vi "ejercicio 3.vi"() -> ()   [LabVIEW 2017]
panel:
  out "numero mayor en renglon":i64[](array[numeric])
  out "suma columnas":i64[](array[numeric])
  out "suma filas":i64[](array[numeric])
  out "renglon\nmax suma":i64
  out "columna\nmax suma":i64
  out "numero mayor\nrenglon 10":i64
  out "numero mayor\nrenglon 9":i64
  out "numero mayor\nrenglon 8":i64
  out "numero mayor\nrenglon 7":i64
  out "numero mayor\nrenglon 6":i64
  out "numero mayor\nrenglon 5":i64
  out "numero mayor\nrenglon 4":i64
  out "numero mayor\nrenglon 3":i64
  out "numero mayor\nrenglon 2":i64
  out "numero mayor\nrenglon 1":i64
  out "Max":i64
  out "Arreglo":i64[][](array[numeric])
  # "Ejercicio 3\nDiseñe un programa que llene una matriz de 10 x 10 y determine:\nEl numero mayor almacenado en la matriz\nEl numero mayor almacenado en cada renglon\nLa columna que tuvo la maxima suma\nEl renglon que tuvo la maxima suma"
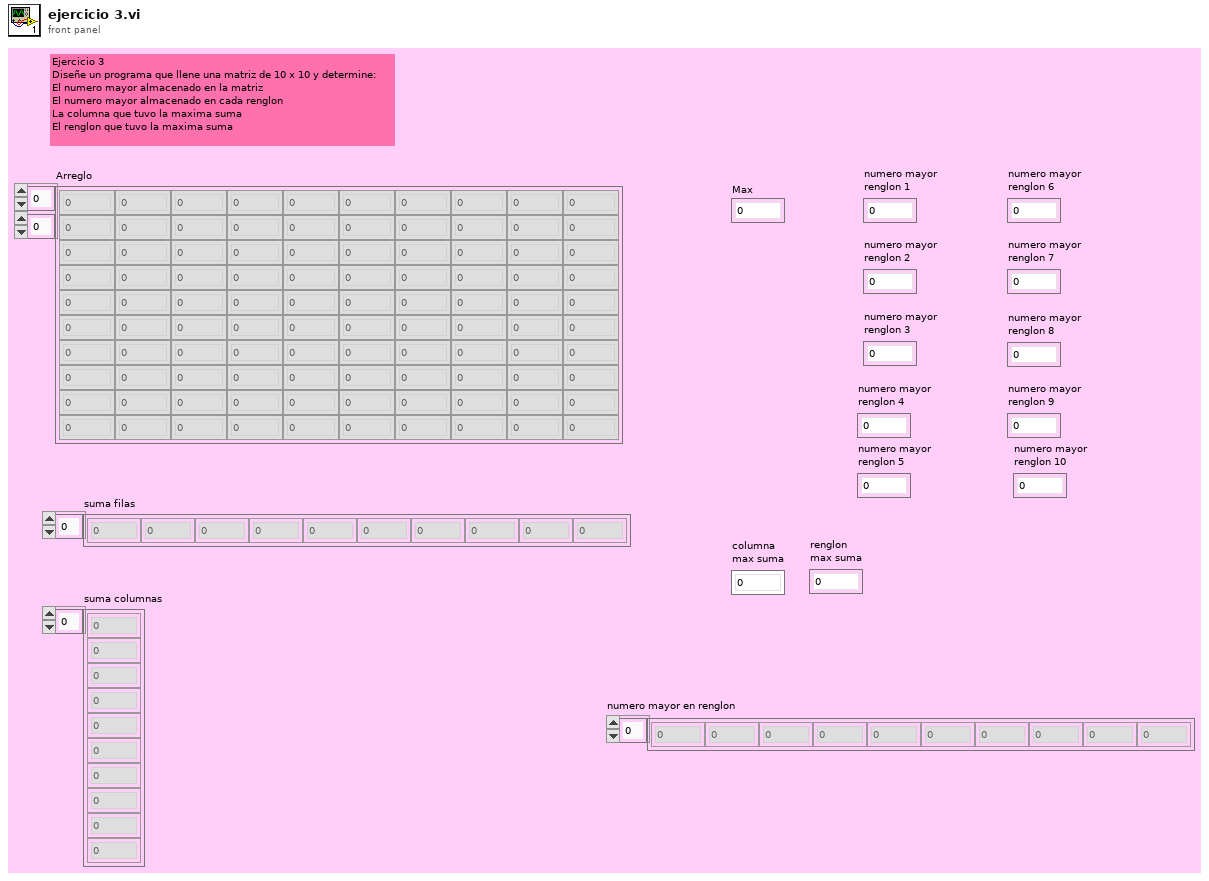
[diagram p1: front panel]
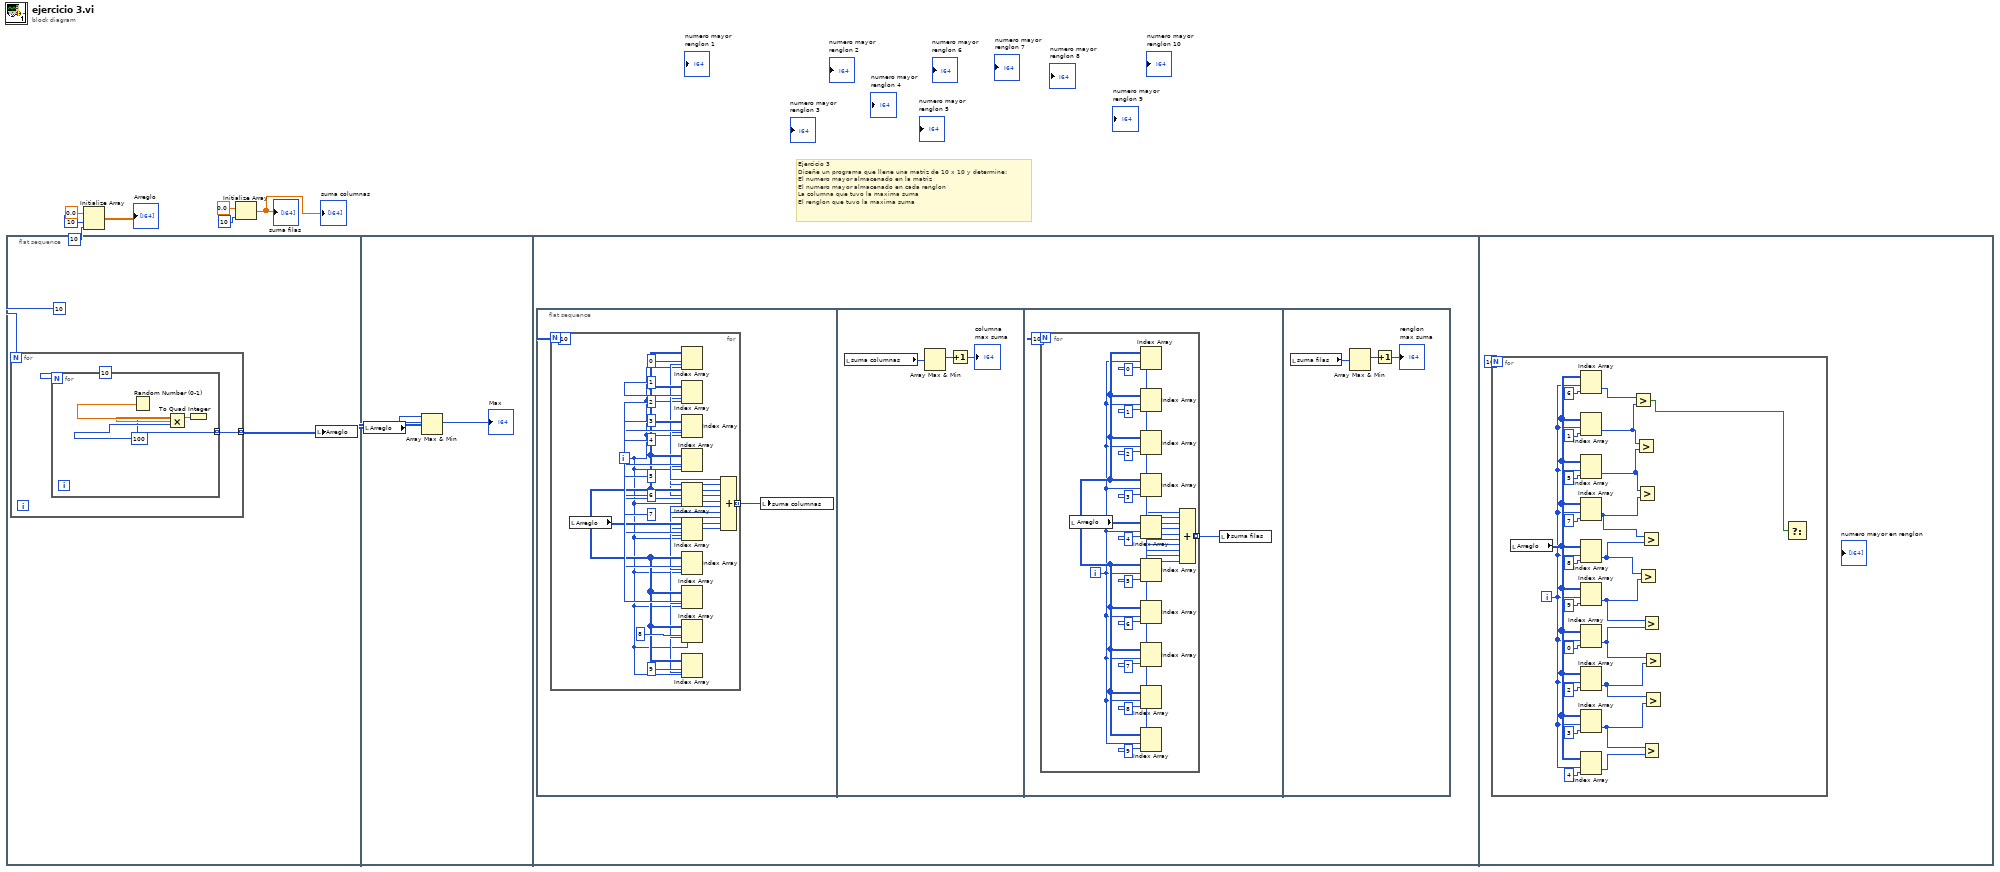
[diagram p0: block diagram]
diagram:
  # "Ejercicio 3\nDiseñe un programa que llene una matriz de 10 x 10 y determine:\nEl numero mayor almacenado en la matriz\nEl numero mayor almacenado en cada renglon\nLa columna que tuvo la maxima suma\nEl renglon que tuvo la maxima suma"
  n1 = flat-sequence {
    frame #0 {
      n2 = for {
        N: 10 ("dimension size") -> [_]
        tunnel: [w10] -> w8 mode=indexing
        n3 = for {
          N: 10 ("dimension size") -> [_]
          tunnel: [w12] -> w10 mode=indexing
          n4 = Random Number (0-1)() -> (number: 0 to 1=w14:dbl)
          n5 = Multiply(x=w14, y=100 ("dimension size")) -> (x*y=w13:dbl)
          n6 = To Quad Integer(1:w13) -> (0:w12:i64)
        }
      }
      n7 = local write "Arreglo"(w8) -> ()
    }
    frame #1 {
      n8 = local read "Arreglo"() -> (w17:i64[][])
      n9 = Array Max & Min(array=w17) -> (max value=→"Max":i64)  [unwired: 3 out]
    }
    frame #2 {
      n10 = flat-sequence {
        frame #0 {
          n11 = for {
            N: 10 -> [_]
            tunnel: [w21] -> w18 mode=indexing
            i -> [w20]
            n12 = local read "Arreglo"() -> (w32:i64[][])
            n13 = Index Array(array=w32, index (row)=0, index (col)=w20) -> (element=w31:i64)
            n14 = Index Array(array=w32, index (row)=1, index (col)=w20) -> (element=w30:i64)
            n15 = Index Array(array=w32, index (row)=2 ("disabled index (col)"), index (col)=w20) -> (element=w29:i64)
            n16 = Index Array(array=w32, index (row)=3 ("disabled index (col)"), index (col)=w20) -> (element=w28:i64)
            n17 = Index Array(array=w32, index (row)=4, index (col)=w20) -> (element=w27:i64)
            n18 = Index Array(array=w32, index (row)=5, index (col)=w20) -> (element=w25:i64)
            n19 = Index Array(array=w32, index (row)=6 ("disabled index (col)"), index (col)=w20) -> (element=w26:i64)
            n20 = Index Array(array=w32, index (row)=7, index (col)=w20) -> (element=w24:i64)
            n21 = Index Array(array=w32, index (row)=8, index (col)=w20) -> (element=w23:i64)
            n22 = Index Array(array=w32, index (row)=9, index (col)=w20) -> (element=w22:i64)
            n23 = Compound Arithmetic op=ADD(w31, w30, w29, w28, w27, w25, w26, w24, w23, w22) -> (w21:i64)
          }
          n24 = local write "suma columnas"(w18) -> ()
        }
        frame #1 {
          n25 = local read "suma columnas"() -> (w45:i64[])
          n26 = Array Max & Min(array=w45) -> (max index (indices)=w44:i32)  [unwired: 3 out]
          n27 = Increment(x=w44) -> (x+1=→"columna\nmax suma":i32)
        }
        frame #2 {
          n28 = for {
            N: 10 -> [_]
            tunnel: [w49] -> w46 mode=indexing
            i -> [w48]
            n29 = local read "Arreglo"() -> (w50:i64[][])
            n30 = Index Array(array=w50, index (row)=w48, index (col)=0 ("disabled index (col)")) -> (element=w61:i64)
            n31 = Index Array(array=w50, index (row)=w48, index (col)=1 ("disabled index (col)")) -> (element=w62:i64)
            n32 = Index Array(array=w50, index (row)=w48, index (col)=2 ("disabled index (col)")) -> (element=w63:i64)
            n33 = Index Array(array=w50, index (row)=w48, index (col)=3 ("disabled index (col)")) -> (element=w64:i64)
            n34 = Index Array(array=w50, index (row)=w48, index (col)=4 ("index (row)")) -> (element=w65:i64)
            n35 = Index Array(array=w50, index (row)=w48, index (col)=5 ("index (row)")) -> (element=w67:i64)
            n36 = Index Array(array=w50, index (row)=w48, index (col)=6 ("disabled index (col)")) -> (element=w66:i64)
            n37 = Index Array(array=w50, index (row)=w48, index (col)=7 ("index (row)")) -> (element=w68:i64)
            n38 = Index Array(array=w50, index (row)=w48, index (col)=8 ("index (row)")) -> (element=w69:i64)
            n39 = Index Array(array=w50, index (row)=w48, index (col)=9 ("index (row)")) -> (element=w70:i64)
            n40 = Compound Arithmetic op=ADD(w61, w62, w63, w64, w65, w67, w66, w68, w69, w70) -> (w49:i64)
          }
          n41 = local write "suma filas"(w46) -> ()
        }
        frame #3 {
          n42 = local read "suma filas"() -> (w72:i64[])
          n43 = Array Max & Min(array=w72) -> (max index (indices)=w73:i32)  [unwired: 3 out]
          n44 = Increment(x=w73) -> (x+1=→"renglon\nmax suma":i32)
        }
      }
    }
    frame #3 {
      n45 = for {
        N: 10 -> [_]
        i -> [w96]
        n46 = local read "Arreglo"() -> (w97:i64[][])
        n47 = Index Array(array=w97, index (row)=w96, index (col)=6 ("disabled index (col)")) -> (element=w85:i64)
        n48 = Index Array(array=w97, index (row)=w96, index (col)=1 ("disabled index (col)")) -> (element=w75:i64)
        n49 = Index Array(array=w97, index (row)=w96, index (col)=5 ("disabled index (col)")) -> (element=w84:i64)
        n50 = Index Array(array=w97, index (row)=w96, index (col)=7 ("disabled index (col)")) -> (element=w83:i64)
        n51 = Index Array(array=w97, index (row)=w96, index (col)=8 ("disabled index (col)")) -> (element=w82:i64)
        n52 = Index Array(array=w97, index (row)=w96, index (col)=9 ("disabled index (col)")) -> (element=w81:i64)
        n53 = Index Array(array=w97, index (row)=w96, index (col)=0 ("disabled index (col)")) -> (element=w80:i64)
        n54 = Index Array(array=w97, index (row)=w96, index (col)=2 ("disabled index (col)")) -> (element=w79:i64)
        n55 = Index Array(array=w97, index (row)=w96, index (col)=3 ("disabled index (col)")) -> (element=w78:i64)
        n56 = Index Array(array=w97, index (row)=w96, index (col)=4 ("disabled index (col)")) -> (element=w77:i64)
        n57 = Greater?(x=w85, y=w75) -> (0:w76:bool)
        n58 = Greater?(x=w75, y=w84) -> ()  [unwired: 1 out]
        n59 = Greater?(x=w84, y=w83) -> ()  [unwired: 1 out]
        n60 = Greater?(x=w82, y=w81) -> ()  [unwired: 1 out]
        n61 = Greater?(x=w83, y=w82) -> ()  [unwired: 1 out]
        n62 = Greater?(x=w81, y=w80) -> ()  [unwired: 1 out]
        n63 = Greater?(x=w78, y=w77) -> ()  [unwired: 1 out]
        n64 = Greater?(x=w80, y=w79) -> ()  [unwired: 1 out]
        n65 = Greater?(x=w79, y=w78) -> ()  [unwired: 1 out]
        n66 = Select(s=w76) -> ()  [unwired: 2 in, 1 out]
      }
    }
  }
  n67 = Initialize Array(0.0 ("element"), 10 ("dimension size"), 10 ("dimension size")) -> (→"Arreglo":dbl[][])
  n68 = Initialize Array(0.0 ("element"), 10 ("dimension size")) -> (→"suma filas" →"suma columnas":dbl[])
